vi "Play Song.vi"(8 "error in (no error)":errorcluster, 10 "Song":refnum<class "Song.lvclass">, 11 "SongPlayerActor in":refnum<class "SongPlayerActor.lvclass">) -> (0 "error out":errorcluster, 3 "SongPlayerActor out":refnum<class "SongPlayerActor.lvclass">)   [LabVIEW 2015, in "SongPlayerActor.lvlib" / "SongPlayerActor.lvclass"]
uses:
  SongPlayerActor.lvclass
  file/MusicElement/Song/Song.lvclass
  SongPlayerActor.lvclass/SongPlayerActor.ctl
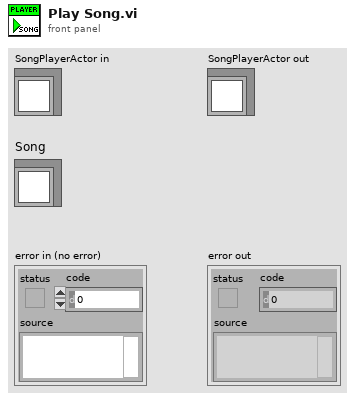
[diagram p1: front panel]
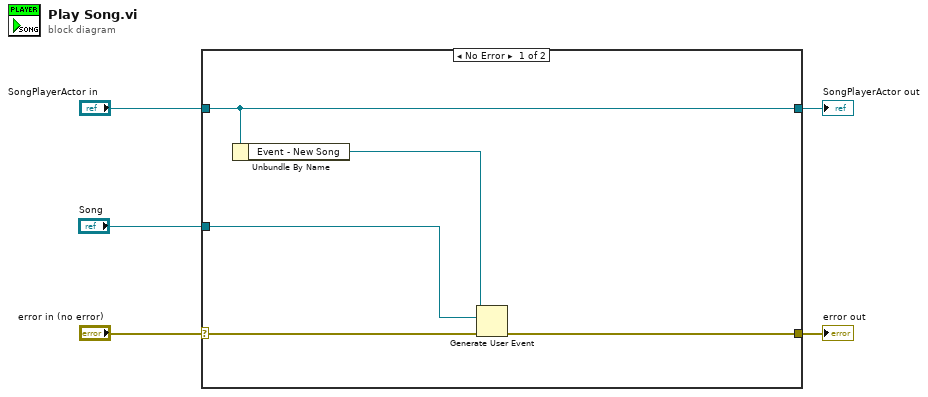
[diagram p0: block diagram]
diagram:
  n1 = case shown="No Error" "error in (no error)" {
    selector: "error in (no error)" -> [w9 w12]
    tunnel: [w6 w12] -> w4
    tunnel: [w10 w11] -> w2
    tunnel: "SongPlayerActor in" -> [w10 w11]
    tunnel: "Song" -> [w7 _]
    frame No Error {
      n2 = Unbundle By Name(w10) -> ("Event - New Song"=w8:refnum<user-event>)
      n3 = Generate User Event(user event=w8, event data cluster=w7, error in=w9) -> (error out=w6:errorcluster)  [unwired: 1 in, 1 out]
    }
    frame Error {
    }
  }
  "error out" <- w4
  "SongPlayerActor out" <- w2
